vi "init_DAC_ao_do_chans.vi"(10 "Rate":dbl=80000.0 format="%#_13g") -> (0 "error out":errorcluster, 3 "AO Out":refnum<k21>, 5 "SampClk.Rate":dbl)   [LabVIEW 2015]
uses:
  <vilib>/DAQmx/create/channels.llb/DAQmx Create Channel (AO-Voltage-Basic).vi
  <vilib>/DAQmx/configure/timing.llb/DAQmx Timing (Sample Clock).vi
  <resource>/objmgr/daqmx.rc
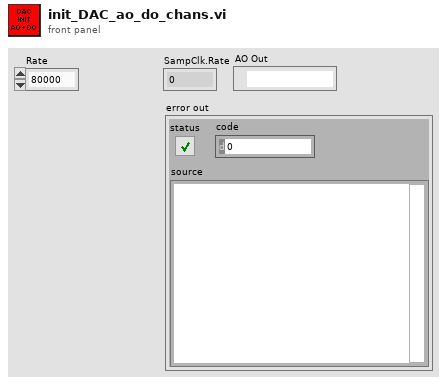
[diagram p1: front panel]
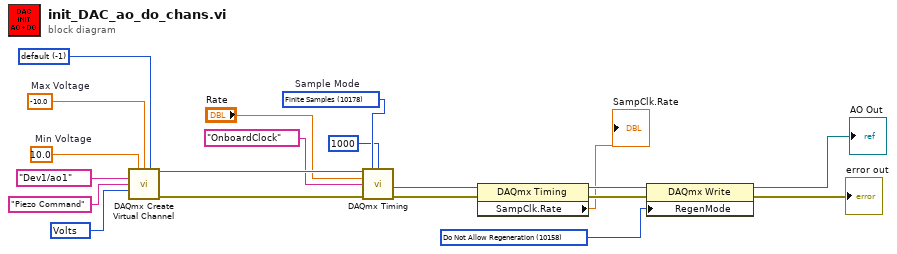
[diagram p0: block diagram]
diagram:
  w20 = 10158 items=["Allow Regeneration"=10097, "Do Not Allow Regeneration"=10158] ("RegenMode")
  w2 = 10178 items=["Finite Samples"=10178, "Continuous Samples"=10123, "Hardware Timed Single Point"=12522]  # Sample Mode
  w13 = -1 items=["default"=-1, "RSE"=10083, "NRSE"=10078, "Differential"=10106, "Pseudodifferential"=12529] ("input terminal configuration")
  w12 = 10348 items=["Volts"=10348, "From Custom Scale"=10065] ("units")
  w8 = 10.0  # Min Voltage
  w9 = -10.0  # Max Voltage
  n1 = call-poly <vilib>:"DAQmx Create Virtual Channel.vi"("maximum value"=w8, "minimum value"=w9, "output terminal configuration"=w13, "physical channels"=tag "Dev1/ao1" ("DAQmx Physical Channel"), "name to assign"="Piezo Command", "units"=w12) -> ("task out"=w6:refnum<k21>, "error out"=w7:errorcluster)  [unwired: 8 in]
  n2 = call-poly <vilib>:"DAQmx Timing.vi"("task/channels in"=w6, "sample mode"=w2, "samples per channel"=1000, "rate"="Rate", "source"=tag "OnboardClock" ("Sample Clock Source"), "error in"=w7) -> ("task out"=w15:refnum<k21>, "error out"=w16:errorcluster)  [unwired: 8 in]
  n3 = property class="DAQmx Timing"(reference=w15, error in=w16) -> (reference out=w17:refnum<k21>, error out=w18:errorcluster, "SampClk.Rate"=→"SampClk.Rate":dbl)
  n4 = property class="DAQmx Write"(reference=w17, error in=w18, "RegenMode"=w20) -> (reference out=→"AO Out":refnum<k21>, error out=→"error out":errorcluster)
